vi "PCtime_Last_Data.vi"() -> ()   [LabVIEW 2012]
panel:
  out "PC time last data":timestamp format="%<%H:%M:%S>T"
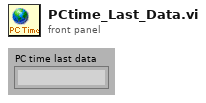
[diagram p1: front panel]
diagram:
